vi "SequenceAquireStreaming.vi"() -> ()   [LabVIEW 2015]
panel:
  out "Intensity Chart":dbl[][](graph)
  in  "Gage Status":bool
  out "size(s)":i32[](array[numeric])
  out "Mode":u16
  out "gage configuration":T1
  in  "abort aquisition":bool
  out "Handle Cluster":T2
  out "Gage status":string
  in  "aquire":bool
  out "current status":T3(ring)
  in  "configure":bool
  in  "Stop Button":bool
  out "error out":errorcluster
  in  "Tab Control":enum32{"aquisition configuration"}(tab)
  in  "streaming":bool
  in  "Sample Rate":dbl=10000000.0
  in  "Zmax":dbl=0.01 format="%#_13g"
  out "aquisition progress":u8(slide) max=1 scale=0.0..100.0
  out "System:":string
  out "system information":T4
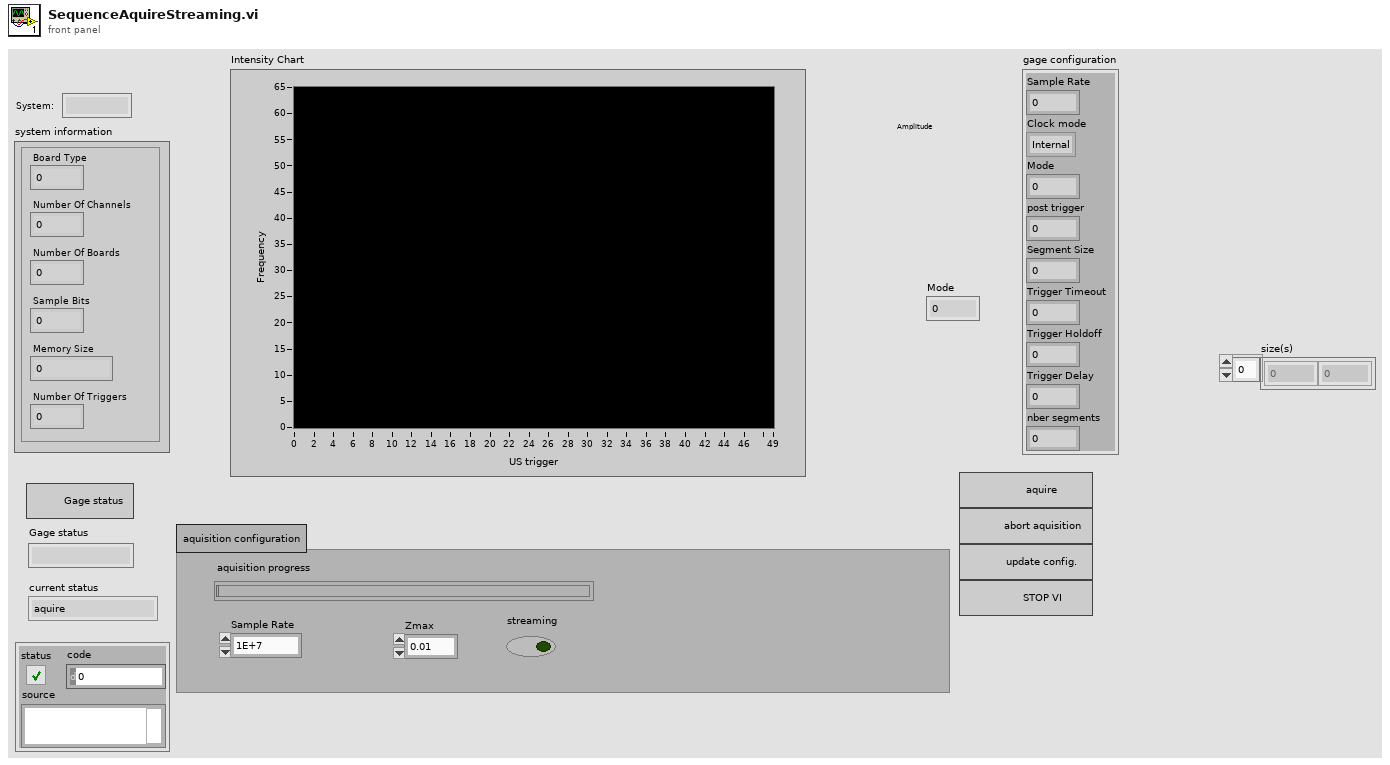
[diagram p1: front panel]
types:
  T1 = cluster{"Sample Rate":dbl, "Clock mode":enum16{"Internal", "External", "Reference"}, "Mode":u16, "post trigger":dbl, "Segment Size":dbl, "Trigger Timeout":dbl, "Trigger Holdoff":dbl, "Trigger Delay":dbl, "nber segments":u32}
  T2 = cluster{"Handle":u32, "Sample size":u32, "Resolution":i32, "Offset":i32, "Channels":u32, "Boards":u32}
  T3 = enum16{"aquire", "configure acquisition", "stop VI", "wait"}
  T4 = cluster{"Memory Size":dbl, "Board Type":u32, "Number Of Channels":u32, "Number Of Boards":u32, "Sample Bits":u32, "Number Of Triggers":u32}
  T5 = cluster{"Slope":u16, "Level":i32, "Source":i32, "External Range":u32, "External Coupling":u16, "External":bool, "Disable":bool, "External Impedance":u16}
  T6 = cluster{"Coupling":u16, "Differential Input":bool, "Direct-to-ADC":bool, "Range":u32, "Impedance":u32, "DC Offset":i32}[]
  T7 = enum16{"aquire", "configure acquisition", "stop VI", "wait"}[]
  T8 = cluster{"Sample Rate":dbl, "Clock mode":enum16{"Internal", "External", "Reference"}, "Mode":u16, "post trigger":dbl, "Segment Size":dbl, "Trigger Timeout":dbl, "Trigger Holdoff":dbl, "Trigger Delay":dbl, "number of records":u32}
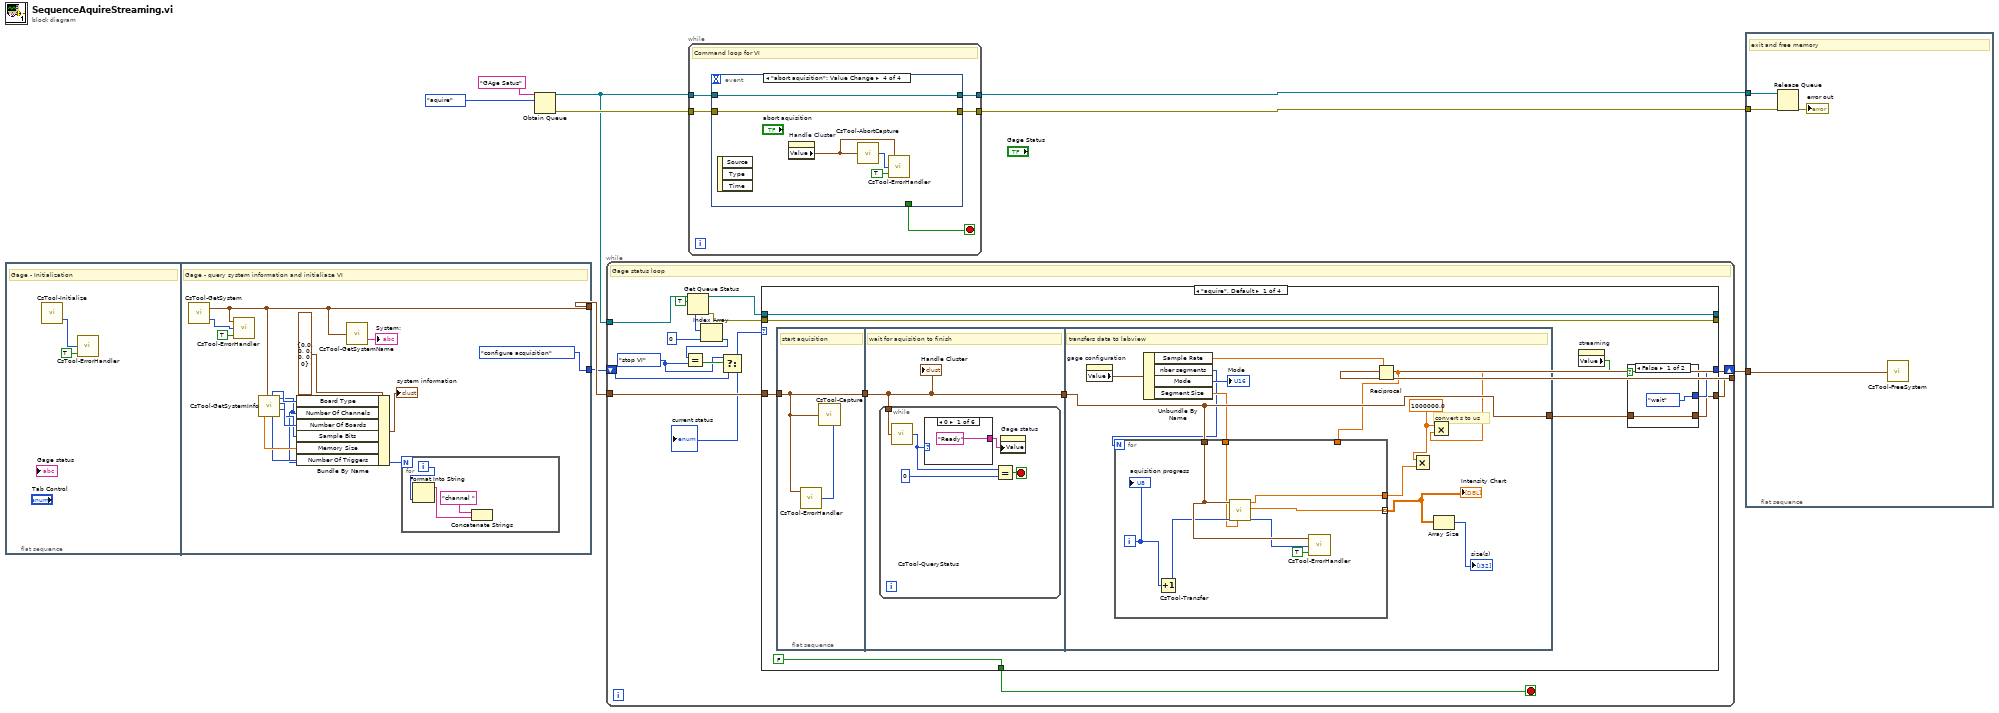
[diagram p0: block diagram]
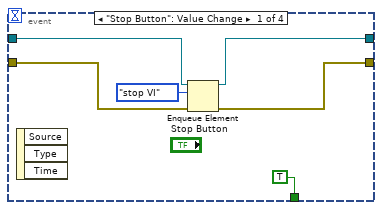
[diagram p2: hidden frame]
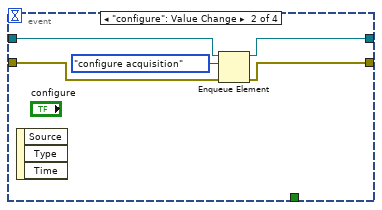
[diagram p3: hidden frame]
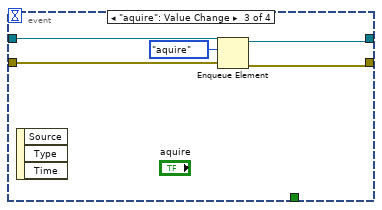
[diagram p4: hidden frame]
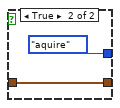
[diagram p5: hidden frame]
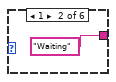
[diagram p6: hidden frame]
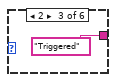
[diagram p7: hidden frame]
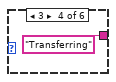
[diagram p8: hidden frame]
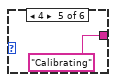
[diagram p9: hidden frame]
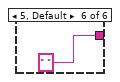
[diagram p10: hidden frame]
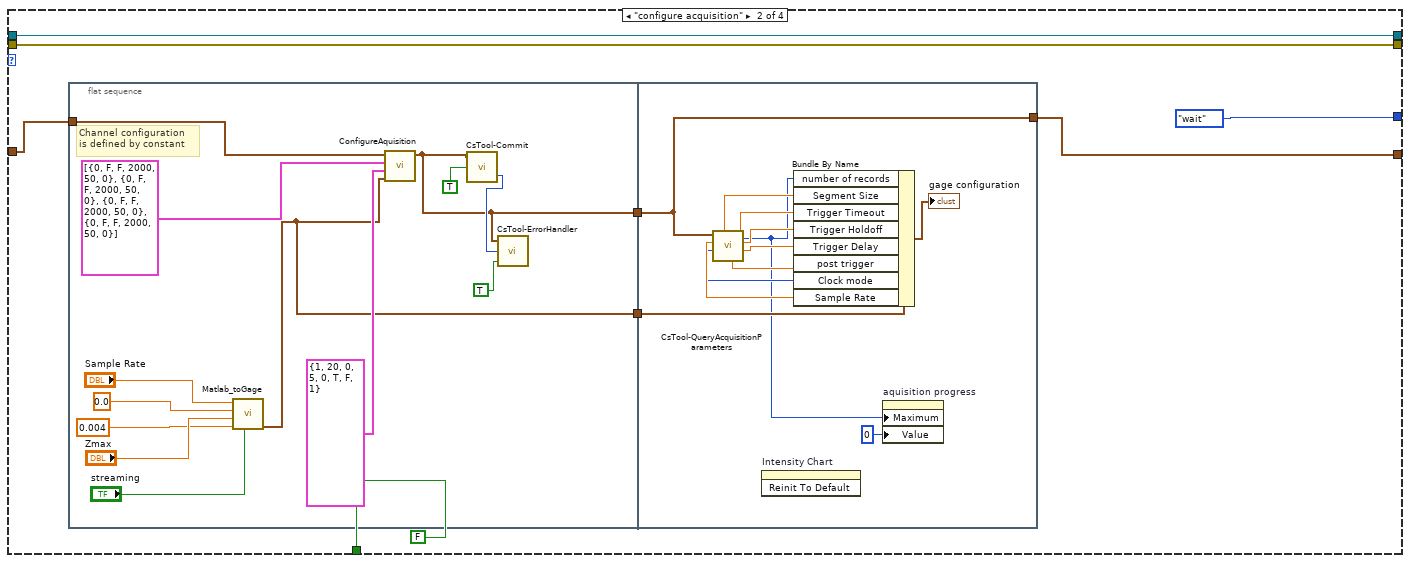
[diagram p11: hidden frame]
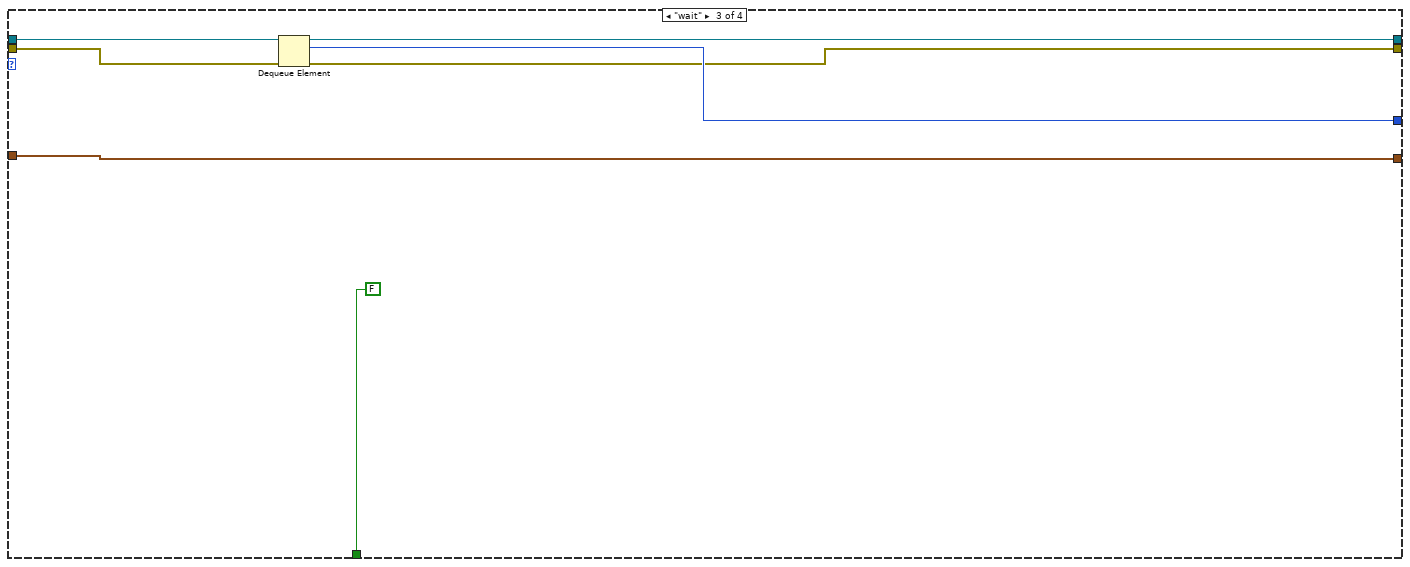
[diagram p12: hidden frame]
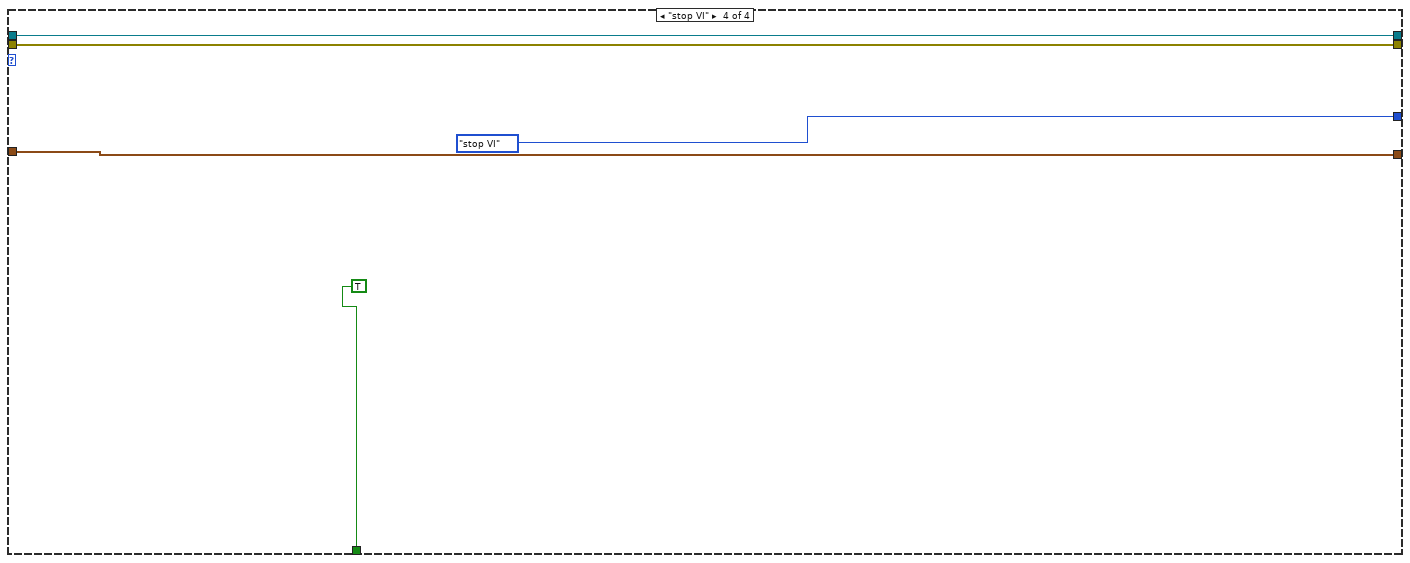
[diagram p13: hidden frame]
diagram:
  n1 = flat-sequence {
    tunnel: [w15] -> w9
    tunnel: [T3."configure acquisition"] -> w1
    frame #0 {
      # "Gage - Initialization"
      n2 = call <userlib>:"CsTool-Initialize.vi"() -> ("Error Code"=w11:i32)  [unwired: 1 out]
      n3 = call <userlib>:"CsTool-ErrorHandler.vi"("StopOnError (true)"=TRUE, "Error Code"=w11) -> ()  [unwired: 1 in, 1 out]
    }
    frame #1 {
      # "Gage - query system information and initialiaze VI"
      n4 = call <userlib>:"CsTool-GetSystem.vi"() -> ("Error Code"=w13:i32, "Handle Cluster"=w15:T2)  [unwired: 4 in]
      n5 = call <userlib>:"CsTool-ErrorHandler.vi"("StopOnError (true)"=TRUE, "Error Code"=w13, "Handle Cluster"=w15) -> ()  [unwired: 1 out]
      n6 = call <userlib>:"CsTool-GetSystemInfo.vi"("Handle Cluster"=w15) -> ("Memory Size"=w21:dbl, "Board Type"=w24:u32, "Number Of Triggers"=w19:u32, "Number Of Channels"=w16:u32, "Number Of Boards"=w23:u32, "Sample Bits"=w22:u32)  [unwired: 1 out]
      n7 = Bundle By Name(cluster=T4 {"Memory Size"=0.0, "Board Type"=0, "Number Of Channels"=0, "Number Of Boards"=0, "Sample Bits"=0, "Number Of Triggers"=0} ("system information"), "Board Type"=w24, "Number Of Channels"=w16, "Number Of Boards"=w23, "Sample Bits"=w22, "Memory Size"=w21, "Number Of Triggers"=w19) -> (→"system information":T4)
      n8 = call <userlib>:"CsTool-GetSystemName.vi"("Handle Cluster"=w15) -> ("System Name"=→"System:":string)  [unwired: 1 out]
      n9 = for {
        N: w16 -> [_]
        i -> [w26]
        n10 = Format Into String(w26) -> (resulting string=w25:string)  [unwired: 3 in, 1 out]
        n11 = Concatenate Strings("channel ", w25) -> ()  [unwired: 1 out]
      }
    }
  }
  n12 = Obtain Queue(name (unnamed)="GAge Satus", element data type=T3."aquire") -> (queue out=w2:refnum<queue>, error out=w6:errorcluster)  [unwired: 3 in, 1 out]
  n13 = while {
    tunnel: w9 -> [w37]
    tunnel: [w36] -> w8
    tunnel: w2 -> [w42]
    shift-right: [w29] -> _
    shift-left: w1 -> [w35]
    stop <- w40 stop-if-true
    w31 = T3."stop VI"
    # "Gage status loop"
    n14 = Get Queue Status(queue=w42, return elements? (F)=TRUE) -> (queue out=w38:refnum<queue>, error out=w28:errorcluster, elements=w41:T7)  [unwired: 1 in, 5 out]
    n15 = Index Array(array=w41, index=0) -> (element=w32:T3)
    n16 = Equal?(x=w32, y=w31) -> (x = y?=w33:bool)
    n17 = Select(t=w31, s=w33, f=w35) -> (s? t:f=w30:T3)
    "current status" <- w30
    n18 = case shown="\"aquire\", Default" w30 {
      tunnel: [FALSE FALSE FALSE TRUE] -> w40
      tunnel: [w51 w96 w127 w133] -> _
      tunnel: w38 -> [w51 w96 w128 w133]
      tunnel: w37 -> [w49 w95 w129 w132]
      tunnel: [w44 w91 w129 w132] -> w36
      tunnel: [w46 T3."wait" w126 T3."stop VI"] -> w29
      tunnel: w28 -> [w50 w93 w125 w130]
      tunnel: [w50 w93 w124 w130] -> _
      frame "aquire", Default {
        n19 = flat-sequence {
          tunnel: w49 -> [w57]
          tunnel: [w57] -> w48
          tunnel: w48 -> [w59]
          tunnel: [w59] -> w47
          tunnel: w47 -> [w81]
          tunnel: [w81] -> w45
          frame #0 {
            # "start aquisition"
            n20 = call <userlib>:"CsTool-Capture.vi"("Handle Cluster"=w57) -> ("Error Code"=w58:i32)
            n21 = call <userlib>:"CsTool-ErrorHandler.vi"("Error Code"=w58, "Handle Cluster"=w57) -> ()  [unwired: 1 in, 1 out]
          }
          frame #1 {
            # "wait for aquisition to finish"
            n22 = while {
              tunnel: w59 -> [w62]
              stop <- w61 stop-if-true
              n23 = call <userlib>:"CsTool-QueryStatus.vi"("Handle Cluster"=w62) -> ("Status"=w64:i32)
              n24 = case shown="0" w64 {
                tunnel: ["Ready" "Waiting" "Triggered" "Transferring" "Calibrating" " "] -> w60
                frame 0 {
                }
                frame 1 {
                }
                frame 2 {
                }
                frame 3 {
                }
                frame 4 {
                }
                frame 5, Default {
                }
              }
              n25 = Equal?(x=w64, y=0) -> (x = y?=w61:bool)
              n26 = property on="Gage status" class="Str"("Value"=w60) -> ()  [unwired: 2 in, 2 out]
            }
            "Handle Cluster" <- w59
          }
          frame #2 {
            w78 = 1000000.0 ("x")
            # "convert s to us"
            # "transfers data to labview"
            n27 = property on="gage configuration" class="Clust (strict)"() -> ("Value"=w77:T1)  [unwired: 2 in, 2 out]
            n28 = Unbundle By Name(w77) -> ("Sample Rate"=w80:dbl, "nber segments"=w72:u32, "Mode"=→"Mode":u16, "Segment Size"=w75:dbl)
            n29 = Reciprocal(x=w80) -> (1/x=w76:dbl)
            n30 = for {
              N: w72 -> [_]
              tunnel: w81 -> [w89]
              tunnel: [w86] -> w79
              tunnel: w76 -> [_]
              tunnel: w75 -> [w84]
              tunnel: [w83] -> w71 mode=indexing
              i -> [w82]
              n31 = Increment(x=w82) -> (x+1=w85:i32)
              n32 = call <userlib>:"CsTool-Transfer.vi"("Length (4096)"=w84, "Segment (1)"=w85, "Handle Cluster"=w89) -> ("Error Code"=w88:i32, "Data in Volts"=w83:dbl[], "Actual Start"=w86:dbl)  [unwired: 3 in, 1 out]
              n33 = call <userlib>:"CsTool-ErrorHandler.vi"("StopOnError (true)"=TRUE, "Error Code"=w88, "Handle Cluster"=w89) -> ()  [unwired: 1 out]
              "aquisition progress" <- w82
            }
            "Intensity Chart" <- w71
            n34 = Multiply(x=w78, y=w79) -> ()  [unwired: 1 out]
            n35 = Multiply(x=w78, y=w76) -> ()  [unwired: 1 out]
            n36 = Array Size(array=w71) -> (size(s)=→"size(s)":i32[])
          }
        }
        n37 = property on="streaming" class="Bool (strict)"() -> ("Value"=w43:bool)  [unwired: 2 in, 2 out]
        n38 = case shown="False" w43 {
          tunnel: [T3."wait" T3."aquire"] -> w46
          tunnel: w45 -> [w53 w55]
          tunnel: [w53 w55] -> w44
          frame False {
          }
          frame True {
          }
        }
      }
      frame "configure acquisition" {
        n39 = flat-sequence {
          tunnel: w95 -> [w110]
          tunnel: [w105] -> w92
          tunnel: [w103] -> w90
          tunnel: [w122] -> w91
          tunnel: w92 -> [w122]
          tunnel: w90 -> [w113]
          frame #0 {
            # "Channel configuration\nis defined by constant"
            n40 = call "Matlab_toGage.vi"("streaming"="streaming", "Xmax"=0.004, "Zmax"="Zmax", "X0"=0.0, "Sample Rate"="Sample Rate") -> ("Acquisition  parameters out"=w103:T8)  [unwired: 6 in]
            n41 = call "ConfigureAquisition.vi"("Acquisition"=w103, "Trigger"=T5 {"Slope"=1, "Level"=20, "Source"=0, "External Range"=5, "External Coupling"=0, "External"=TRUE, "Disable"=FALSE, "External Impedance"=1}, "channels configuration"=T6 [{"Coupling"=0, "Differential Input"=FALSE, "Direct-to-ADC"=FALSE, "Range"=2000, "Impedance"=50, "DC Offset"=0}, {"Coupling"=0, "Differential Input"=FALSE, "Direct-to-ADC"=FALSE, "Range"=2000, "Impedance"=50, "DC Offset"=0}, {"Coupling"=0, "Differential Input"=FALSE, "Direct-to-ADC"=FALSE, "Range"=2000, "Impedance"=50, "DC Offset"=0}, {"Coupling"=0, "Differential Input"=FALSE, "Direct-to-ADC"=FALSE, "Range"=2000, "Impedance"=50, "DC Offset"=0}] ("channels \nconfiguration"), "Handle Cluster"=w110) -> ("Handle Cluster 2"=w105:T2)  [unwired: 6 in, 1 out]
            n42 = call <userlib>:"CsTool-Commit.vi"("Coerce Flag (f)"=TRUE, "Handle Cluster"=w105) -> ("Error Code"=w106:i32)  [unwired: 1 in, 1 out]
            n43 = call <userlib>:"CsTool-ErrorHandler.vi"("StopOnError (true)"=TRUE, "Error Code"=w106, "Handle Cluster"=w105) -> ()  [unwired: 1 out]
          }
          frame #1 {
            n44 = call <userlib>:"CsTool-QueryAcquisitionParameters.vi"("Handle Cluster"=w122) -> ("Trigger Delay"=w118:dbl, "Trigger Holdoff"=w117:dbl, "Trigger Timeout"=w116:dbl, "Depth"=w119:dbl, "Segment Count"=w112:u32, "Segment Size"=w115:dbl, "Clock Mode"=w120:enum16{"Internal", "External", "Reference"}, "Sample Rate"=w121:dbl)  [unwired: 3 out]
            n45 = invoke on="Intensity Chart" class="IntChart (strict)" method="Reinit To Default"() -> ()  [unwired: 3 in, 3 out]
            n46 = Bundle By Name(cluster=w113, "number of records"=w112, "Segment Size"=w115, "Trigger Timeout"=w116, "Trigger Holdoff"=w117, "Trigger Delay"=w118, "post trigger"=w119, "Clock mode"=w120, "Sample Rate"=w121) -> (→"gage configuration":T8)
            n47 = property on="aquisition progress" class="Slide (strict)"("Maximum"=w112, "Value"=u8 0 ("aquisition progress")) -> ()  [unwired: 2 in, 2 out]
          }
        }
      }
      frame "wait" {
        n48 = Dequeue Element(queue=w128, error in (no error)=w125) -> (queue out=w127:refnum<queue>, element=w126:T3, error out=w124:errorcluster)  [unwired: 1 in, 1 out]
      }
      frame "stop VI" {
      }
    }
  }
  n49 = while {
    tunnel: w6 -> [w138]
    tunnel: w2 -> [w139]
    tunnel: [w137] -> w4
    tunnel: [w136] -> w3
    stop <- w135 stop-if-true
    # "Command loop for VI"
    n50 = event shown="[3] \"abort aquisition\": Value Change" {
      selector: _ -> [_ _ _ _]
      dyn-events: _ -> [_ _ _ _]
      timeout: _ -> [_ _ _ _]
      tunnel: w139 -> [w145 w150 w155 w159]
      tunnel: w138 -> [w144 w147 w153 w160]
      tunnel: [w142 w149 w154 w159] -> w137
      tunnel: [w141 w148 w152 w160] -> w136
      tunnel: [TRUE _ _ _] -> w135
      event "Stop Button": Value Change {
        n51 = event-data() -> ()  [unwired: 1 in, 3 out]
        n52 = Enqueue Element(queue=w145, element=T3."stop VI", error in (no error)=w144) -> (queue out=w142:refnum<queue>, error out=w141:errorcluster)  [unwired: 1 in, 1 out]
      }
      event "configure": Value Change {
        n53 = event-data() -> ()  [unwired: 1 in, 3 out]
        n54 = Enqueue Element(queue=w150, element=T3."configure acquisition", error in (no error)=w147) -> (queue out=w149:refnum<queue>, error out=w148:errorcluster)  [unwired: 1 in, 1 out]
      }
      event "aquire": Value Change {
        n55 = event-data() -> ()  [unwired: 1 in, 3 out]
        n56 = Enqueue Element(queue=w155, element=T3."aquire", error in (no error)=w153) -> (queue out=w154:refnum<queue>, error out=w152:errorcluster)  [unwired: 1 in, 1 out]
      }
      event "abort aquisition": Value Change {
        n57 = event-data() -> ()  [unwired: 1 in, 3 out]
        n58 = property on="Handle Cluster" class="Clust (strict)"() -> ("Value"=w157:T2)  [unwired: 2 in, 2 out]
        n59 = call <userlib>:"CsTool-AbortCapture.vi"("Handle Cluster"=w157) -> ("Error Code"=w158:i32)
        n60 = call <userlib>:"CsTool-ErrorHandler.vi"("StopOnError (true)"=TRUE, "Error Code"=w158, "Handle Cluster"=w157) -> ()  [unwired: 1 out]
      }
    }
  }
  n61 = flat-sequence {
    tunnel: w8 -> [w164]
    tunnel: w4 -> [w163]
    tunnel: w3 -> [w162]
    frame #0 {
      # "exit and free memory"
      n62 = Release Queue(queue=w163, error in (no error)=w162) -> (error out=→"error out":errorcluster)  [unwired: 1 in, 2 out]
      n63 = call <userlib>:"CsTool-FreeSystem.vi"("Handle Cluster"=w164) -> ()  [unwired: 1 out]
    }
  }
